vi "binary record both ch.vi"(3 "xIncrement":dbl, 4 "Record":bool, 5 "gain":dbl=1.0, 6 "offset":dbl, 7 "relativeInitialX":dbl, 8 "Index files\npath array":i32, 9 "Files path array":path[](array[path]), 10 "wfm":i16[][](array[numeric]), 11 "reference":refnum<vi>) -> ()   [LabVIEW 2013]
panel:
  out "error out":errorcluster
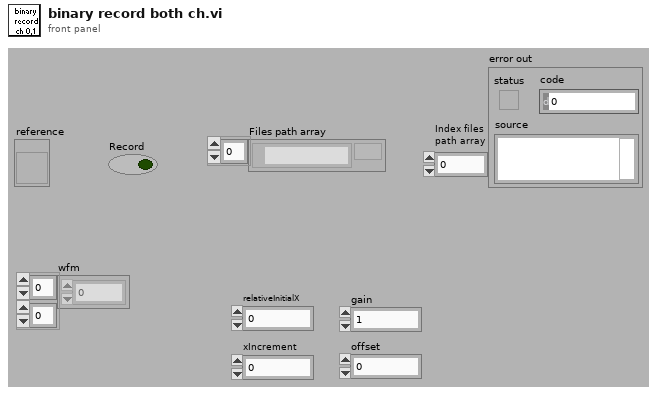
[diagram p1: front panel]
types:
  T1 = enum16{"open", "replace", "create", "open or create", "replace or create", "replace or create with confirmation"}
  T2 = enum16{"big-endian, network order", "native, host order", "little-endian"}
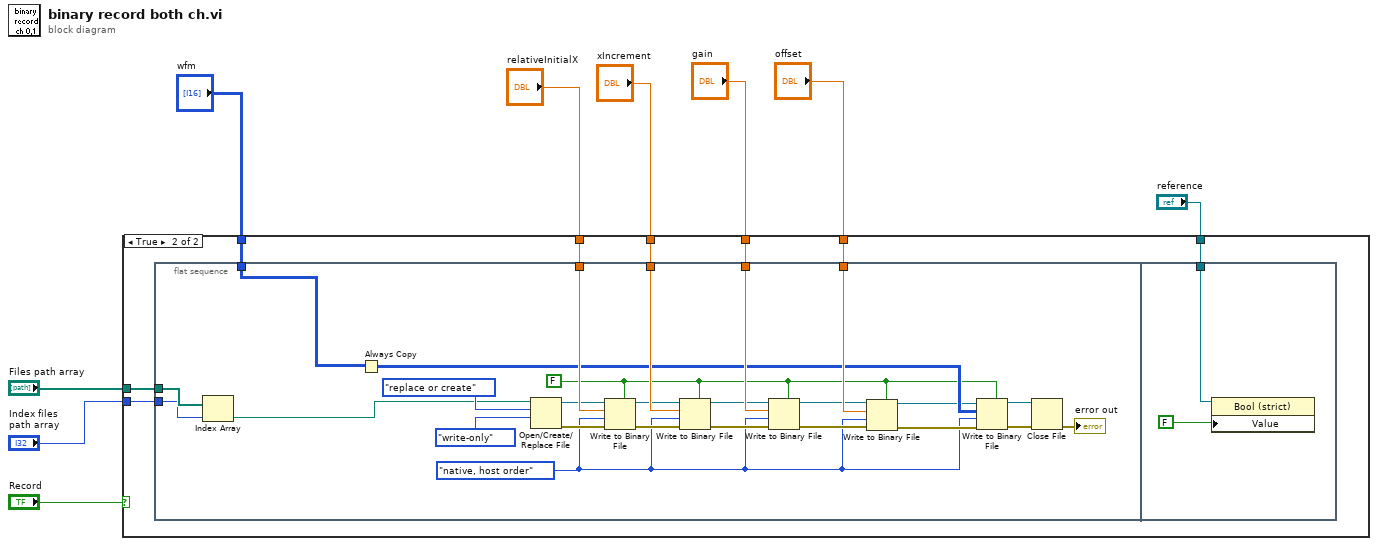
[diagram p0: block diagram]
diagram:
  n1 = case shown="True" "Record" {
    tunnel: "wfm" -> [_ w17]
    tunnel: "relativeInitialX" -> [_ w16]
    tunnel: "xIncrement" -> [_ w15]
    tunnel: "gain" -> [_ w14]
    tunnel: "offset" -> [_ w13]
    tunnel: "reference" -> [_ w12]
    tunnel: "Files path array" -> [_ w11]
    tunnel: "Index files\npath array" -> [_ w10]
    frame False {
    }
    frame True {
      n2 = flat-sequence {
        tunnel: w17 -> [w19]
        tunnel: w16 -> [w43]
        tunnel: w15 -> [w42]
        tunnel: w14 -> [w41]
        tunnel: w13 -> [w40]
        tunnel: w11 -> [w21]
        tunnel: w10 -> [w20]
        tunnel: w12 -> [w44]
        frame #0 {
          w23 = FALSE ("prepend array or string size? (T)")
          w24 = T2."native, host order" ("byte order (0:big-endian, network order)")
          n3 = Index Array(array=w21, index=w20) -> (element=w22:path)
          n4 = Always Copy(1:w19) -> (0:w37:i16[][])
          n5 = Open/Create/Replace File(file path (use dialog)=w22, operation (0:open)=T1."replace or create", access (0:read/write)=enum16{"read/write", "read-only", "write-only"}."write-only") -> (refnum out=w36:refnum<file>, error out=w35:errorcluster)  [unwired: 1 in, 3 out]
          n6 = Write to Binary File(file (use dialog)=w36, data=w43, error in=w35, 5:w23, 9:w24) -> (refnum out=w34:refnum<file>, error out=w33:errorcluster)  [unwired: 2 out]
          n7 = Write to Binary File(file (use dialog)=w34, data=w42, error in=w33, 5:w23, 9:w24) -> (refnum out=w32:refnum<file>, error out=w28:errorcluster)  [unwired: 2 out]
          n8 = Write to Binary File(file (use dialog)=w32, data=w41, error in=w28, 5:w23, 9:w24) -> (refnum out=w31:refnum<file>, error out=w27:errorcluster)  [unwired: 2 out]
          n9 = Write to Binary File(file (use dialog)=w31, data=w40, error in=w27, 5:w23, 9:w24) -> (refnum out=w30:refnum<file>, error out=w26:errorcluster)  [unwired: 2 out]
          n10 = Write to Binary File(file (use dialog)=w30, data=w37, error in=w26, 5:w23, 9:w24) -> (refnum out=w29:refnum<file>, error out=w25:errorcluster)  [unwired: 2 out]
          n11 = Close File(refnum=w29, error in=w25) -> (error out=→"error out":errorcluster)  [unwired: 1 out]
        }
        frame #1 {
          n12 = property on="Property Node" class="Bool (strict)"(reference=w44, "Value"=FALSE ("Boolean")) -> ()  [unwired: 1 in, 2 out]
        }
      }
    }
  }
